vi "Test2_3a_ASIC.vi"(1 "Att. Gain":i32[](array[numeric])=[0, 15], 4 "Voltages comprobation":dbl[](array[numeric])=[0.05, 0.1, 0.2, 0.5, 0.8], 5 "Serial number":string="SN002", 6 "IB_Clip":i32[](array[numeric])=[7, 31, 63], 7 "Save NOW!":bool, 8 "error in":errorcluster, 9 "Cycles Burst":i32=10000, 10 "Channels":i32[](array[numeric])=[0, 1, 2, 3, 4, 5, 6], 11 "Instrument VISA in":T1={"AWG VISA"="generadorpulsos", "Oscilloscope  VISA "="Oscilloscope", "Integration Board IP"="172.16.7.43", "connection ID"=refnum, "report out"=refnum, "report file path"=path "C:/Documents and Settings/CTA_LAB01/Desktop/L0_Asic/L0 Asic Test Data"}) -> (0 "error out":errorcluster={"status"=TRUE, "code"=-1074000000, "source"="Agilent 8000 Series.lvlib:Error Query.vi<ERR>\nInstrument reports:\n-410,\"Query INTERRUPTED\"\r\n0,\"No error\"\r\n\n\n\n<b>Complete call chain:</b>\r\n     Agilent 8000 Series.lvlib:Error Query.vi\r\n     Agilent 8000 Series.lvlib:Close.vi\r\n     Test2_3a_ASIC.vi\r\n     Test_Sum_plus_Maj.vi"}, 3 "Instrument VISA out":T1={"AWG VISA"="generadorpulsos", "Oscilloscope  VISA "="Oscilloscope", "Integration Board IP"="172.16.7.43", "connection ID"=refnum, "report out"=refnum, "report file path"=path "C:/Documents and Settings/CTA_LAB01/Desktop/L0_Asic/L0 Asic Test Data"})   [LabVIEW 2009]
uses:
  <vilib>/Utility/NIReport.llb/NI_report.lvclass
  <vilib>/Utility/NIReport.llb/HTML/NI_HTML.lvclass
  L0_Asic/L0 Asic Test Folder v9/C/Program Files/National Instruments/LabVIEW 2012/instr.lib/Agilent 8000 Series/Public/Configure/Configure Math (Binary Operation).vi
  <instrlib>/Agilent 8000 Series/Public/Data/Read (Multiple Waveforms).vi
  <instrlib>/Agilent 81150/Agilent 81150.lvlib
  L0_Asic/L0 Asic Test Folder v9/C/Program Files/National Instruments/LabVIEW 2012/instr.lib/Agilent 8000 Series/Agilent 8000 Series.lvlib
panel:
  out "dt":dbl
  out "report file path":path=path "C:/Documents and Settings/CTA_LAB01/Desktop/L0_Asic/L0 Asic Test Data"
  in  "Full waveform":bool
  out "Waveform Data":waveform(dbl)[](graph)
  out "time for channel bucle":u32=4294966932
  out "iindex inner bucle":u16=36
  out "time attenuation bucle":u32
  out "points quantity":dbl=10.0
  out "appended array":dbl[](array[numeric])=[9.99999e+37, 9.99999e+37, 2.123674e-09, 7.3101e-11, 0.039346, 0.000993, 2.289694e-09, 1.06004e-10, 1.2407375e-08, 6.2001e-11, 10.0]
  out "read buffer 3":string="V amptd(1),9.99999E+37,9.99999E+37,9.99999E+37,9.99999E+37,9.99999E+37,1.0E+01,+ width(1),2.01719E-09,1.96859E-09,2.19026E-09,2.123674E-09,7.3101E-11,1.0E+01,V amptd(f2),4.065E-02,3.735E-02,4.065E-02,3.9346E-02,9.93E-04,1.0E+01,+ width(f2),2.36565E-09,2.08540E-09,2.47853E-09,2.289694E-09,1.06004E-10,1.0E+01,Time(1-f2),1.236997E-08,1.232364E-08,1.250940E-08,1.2407375E-08,6.2001E-11,1.0E+01\n"
  out "bucle for inner bucle":u32=807
  out "Numeric":i32=185157552
  in  "Clip_sel_b":u32
  in  "Quantity of measurements":u32=100
  in  "End 2":bool
  out "Data output":dbl[][](array[numeric])=[[0.05, 0.0, 0.0, 63.0, 1.0, 9.99999e+37, 9.99999e+37, 2.153239e-09, 8.9127e-11, 0.042394, 0.001347, 2.171806e-09, 1.11555e-10, 1.245617e-08, 7.5484e-11, 10.0, 0.0784, 0.008304761904761905, 0.0], [0.05, 0.0, 0.0, 61.0, 1.0, 9.99999e+37, 9.99999e+37, 2.17591e-09, 7.5138e-11, 0.040364, 0.001353, 2.209888e-09, 7.8523e-11, 1.2524514e-08, 6.7029e-11, 10.0, 0.0784, 0.008304761904761905, 1.0], [0.05, 0.0, 0.0, 59.0, 1.0, 9.99999e+37, 9.99999e+37, 2.193132e-09, 9.3873e-11, 0.04121, 0.001373, 2.164955e-09, 7.7804e-11, 1.2473393e-08, 1.08096e-10, 10.0, 0.0784, 0.008304761904761905, 2.0], [0.05, 0.0, 0.0, 57.0, 1.0, 9.99999e+37, 9.99999e+37, 2.180741e-09, 4.2203e-11, 0.041548, 0.002229, 2.169974e-09, 9.3751e-11, 1.2444116e-08, 5.5272e-11, 11.0, 0.0784, 0.008304761904761905, 3.0], [0.05, 0.0, 0.0, 55.0, 1.0, 9.99999e+37, 9.99999e+37, 2.11229e-09, 3.944e-11, 0.04008, 0.00163, 2.2755e-09, 8.158e-11, 1.245845e-08, 6.277e-11, 9.0, 0.0784, 0.008304761904761905, 4.0], [0.05, 0.0, 0.0, 53.0, 1.0, 9.99999e+37, 9.99999e+37, 2.155237e-09, 6.5891e-11, 0.041291, 0.001559, 2.232596e-09, 7.6359e-11, 1.2466949e-08, 7.7547e-11, 10.0, 0.0784, 0.008304761904761905, 5.0], [0.05, 0.0, 0.0, 7.0, 1.0, 9.99999e+37, 9.99999e+37, 2.12755e-09, 9.1771e-11, 0.03769, 0.001358, 2.349888e-09, 1.38811e-10, 1.2670959e-08, 9.0849e-11, 11.0, 0.0784, 0.008304761904761905, 6.0], [0.05, 0.0, 0.0, 31.0, 1.0, 9.99999e+37, 9.99999e+37, 2.125787e-09, 6.702e-11, 0.039923, 0.00164, 2.260289e-09, 8.9941e-11, 1.2540436e-08, 8.3431e-11, 10.0, 0.0784, 0.008304761904761905, 7.0], [0.05, 0.0, 0.0, 63.0, 1.0, 9.99999e+37, 9.99999e+37, 2.197528e-09, 1.15595e-10, 0.040956, 0.001571, 2.140684e-09, 8.7113e-11, 1.2455007e-08, 4.6485e-11, 10.0, 0.0784, 0.008304761904761905, 8.0], [0.05, 1.0, 0.0, 63.0, 1.0, 9.99999e+37, 9.99999e+37, 2.162133e-09, 7.0698e-11, 0.041207, 0.000752, 2.208266e-09, 1.00999e-10, 1.2372613e-08, 1.00276e-10, 10.0, 0.0784, 0.008304761904761905, 9.0], [0.05, 1.0, 0.0, 61.0, 1.0, 9.99999e+37, 9.99999e+37, 2.13661e-09, 8.2189e-11, 0.039983, 0.00187, 2.265451e-09, 1.14003e-10, 1.2402013e-08, 7.7045e-11, 10.0, 0.0784, 0.008304761904761905, 10.0], [0.05, 1.0, 0.0, 59.0, 1.0, 9.99999e+37, 9.99999e+37, 2.141268e-09, 1.12814e-10, 0.039793, 0.001662, 2.269538e-09, 1.06589e-10, 1.2427868e-08, 8.2834e-11, 10.0, 0.0784, 0.008304761904761905, 11.0], [0.05, 1.0, 0.0, 57.0, 1.0, 9.99999e+37, 9.99999e+37, 2.049403e-09, 8.9792e-11, 0.039527, 0.002147, 2.280746e-09, 1.28958e-10, 1.2384183e-08, 7.0735e-11, 10.0, 0.0784, 0.008304761904761905, 12.0], [0.05, 1.0, 0.0, 55.0, 1.0, 9.99999e+37, 9.99999e+37, 2.164408e-09, 7.8869e-11, 0.041681, 0.001876, 2.182885e-09, 9.6951e-11, 1.2340938e-08, 7.1672e-11, 11.0, 0.0784, 0.008304761904761905, 13.0], [0.05, 1.0, 0.0, 53.0, 1.0, 9.99999e+37, 9.99999e+37, 2.181125e-09, 8.9741e-11, 0.040692, 0.002137, 2.217623e-09, 7.9633e-11, 1.2395418e-08, 1.04033e-10, 10.0, 0.0784, 0.008304761904761905, 14.0], [0.05, 1.0, 0.0, 7.0, 1.0, 9.99999e+37, 9.99999e+37, 2.09233e-09, 6.5939e-11, 0.038027, 0.002128, 2.292623e-09, 1.35118e-10, 1.2538524e-08, 8.874e-11, 10.0, 0.0784, 0.008304761904761905, 15.0], [0.05, 1.0, 0.0, 31.0, 1.0, 9.99999e+37, 9.99999e+37, 2.195349e-09, 8.3233e-11, 0.041018, 0.002034, 2.227655e-09, 8.0651e-11, 1.2425997e-08, 6.1393e-11, 10.0, 0.0784, 0.008304761904761905, 16.0], [0.05, 1.0, 0.0, 63.0, 1.0, 9.99999e+37, 9.99999e+37, 2.150328e-09, 1.0069e-10, 0.040933, 0.00205, 2.19783e-09, 8.0511e-11, 1.2358424e-08, 7.9804e-11, 11.0, 0.0784, 0.008304761904761905, 17.0], [0.05, 2.0, 0.0, 63.0, 1.0, 9.99999e+37, 9.99999e+37, 2.146071e-09, 1.27898e-10, 0.040824, 0.001718, 2.206733e-09, 8.1062e-11, 1.2336427e-08, 5.726e-11, 10.0, 0.0784, 0.008304761904761905, 18.0], [0.05, 2.0, 0.0, 61.0, 1.0, 9.99999e+37, 9.99999e+37, 2.18257e-09, 8.9257e-11, 0.040006, 0.001447, 2.192466e-09, 1.10596e-10, 1.2368096e-08, 6.3926e-11, 10.0, 0.0784, 0.008304761904761905, 19.0], [0.05, 2.0, 0.0, 59.0, 1.0, 9.99999e+37, 9.99999e+37, 2.127276e-09, 7.6459e-11, 0.040334, 0.001234, 2.248995e-09, 1.01211e-10, 1.2365757e-08, 3.5637e-11, 10.0, 0.0784, 0.008304761904761905, 20.0], [0.05, 2.0, 0.0, 57.0, 1.0, 9.99999e+37, 9.99999e+37, 2.126691e-09, 1.01851e-10, 0.041905, 0.001534, 2.214677e-09, 1.14645e-10, 1.2361141e-08, 9.1969e-11, 10.0, 0.0784, 0.008304761904761905, 21.0], [0.05, 2.0, 0.0, 55.0, 1.0, 9.99999e+37, 9.99999e+37, 2.192435e-09, 9.9832e-11, 0.040764, 0.00096, 2.19804e-09, 6.5482e-11, 1.2364743e-08, 9.3874e-11, 10.0, 0.0784, 0.008304761904761905, 22.0], [0.05, 2.0, 0.0, 53.0, 1.0, 9.99999e+37, 9.99999e+37, 2.153844e-09, 6.2552e-11, 0.039026, 0.001388, 2.246022e-09, 9.7907e-11, 1.2344355e-08, 4.8187e-11, 10.0, 0.0784, 0.008304761904761905, 23.0], [0.05, 2.0, 0.0, 7.0, 1.0, 9.99999e+37, 9.99999e+37, 2.218394e-09, 8.2589e-11, 0.037653, 0.001409, 2.315577e-09, 9.9529e-11, 1.2540865e-08, 5.8072e-11, 10.0, 0.0784, 0.008304761904761905, 24.0], [0.05, 2.0, 0.0, 31.0, 1.0, 9.99999e+37, 9.99999e+37, 2.142179e-09, 6.129e-11, 0.040237, 0.001325, 2.255953e-09, 8.6753e-11, 1.2411504e-08, 8.6298e-11, 10.0, 0.0784, 0.008304761904761905, 25.0], [0.05, 2.0, 0.0, 63.0, 1.0, 9.99999e+37, 9.99999e+37, 2.16678e-09, 7.307e-11, 0.03966, 0.00193, 2.25843e-09, 1.2459e-10, 1.238779e-08, 9.08e-11, 9.0, 0.0784, 0.008304761904761905, 26.0], [0.05, 3.0, 0.0, 63.0, 1.0, 9.99999e+37, 9.99999e+37, 2.121706e-09, 9.3892e-11, 0.039916, 0.001529, 2.262652e-09, 7.8947e-11, 1.2388872e-08, 8.2672e-11, 10.0, 0.0784, 0.008304761904761905, 27.0], [0.05, 3.0, 0.0, 61.0, 1.0, 9.99999e+37, 9.99999e+37, 2.182719e-09, 9.6917e-11, 0.038637, 0.001642, 2.243077e-09, 1.01628e-10, 1.2393225e-08, 7.9278e-11, 11.0, 0.0784, 0.008304761904761905, 28.0], [0.05, 3.0, 0.0, 59.0, 1.0, 9.99999e+37, 9.99999e+37, 2.104882e-09, 7.8145e-11, 0.039545, 0.001416, 2.260672e-09, 6.9312e-11, 1.2373319e-08, 5.982e-11, 10.0, 0.0784, 0.008304761904761905, 29.0], [0.05, 3.0, 0.0, 57.0, 1.0, 9.99999e+37, 9.99999e+37, 2.143059e-09, 1.1147e-10, 0.039547, 0.001283, 2.287147e-09, 7.9568e-11, 1.2389127e-08, 5.2602e-11, 11.0, 0.0784, 0.008304761904761905, 30.0], [0.05, 3.0, 0.0, 55.0, 1.0, 9.99999e+37, 9.99999e+37, 2.10482e-09, 6.9561e-11, 0.039043, 0.00127, 2.273205e-09, 8.8457e-11, 1.2378439e-08, 8.4875e-11, 10.0, 0.0784, 0.008304761904761905, 31.0], [0.05, 3.0, 0.0, 53.0, 1.0, 9.99999e+37, 9.99999e+37, 2.166631e-09, 9.2658e-11, 0.039151, 0.000816, 2.302048e-09, 1.32139e-10, 1.2463216e-08, 8.3773e-11, 10.0, 0.0784, 0.008304761904761905, 32.0], [0.05, 3.0, 0.0, 7.0, 1.0, 9.99999e+37, 9.99999e+37, 2.098564e-09, 6.1759e-11, 0.037315, 0.001398, 2.363454e-09, 7.7253e-11, 1.2590485e-08, 6.8209e-11, 10.0, 0.0784, 0.008304761904761905, 33.0], [0.05, 3.0, 0.0, 31.0, 1.0, 9.99999e+37, 9.99999e+37, 2.135125e-09, 7.3789e-11, 0.03888, 0.001329, 2.298536e-09, 5.3729e-11, 1.2501362e-08, 7.0595e-11, 10.0, 0.0784, 0.008304761904761905, 34.0], [0.05, 3.0, 0.0, 63.0, 1.0, 9.99999e+37, 9.99999e+37, 2.123674e-09, 7.3101e-11, 0.039346, 0.000993, 2.289694e-09, 1.06004e-10, 1.2407375e-08, 6.2001e-11, 10.0, 0.0784, 0.008304761904761905, 35.0]]
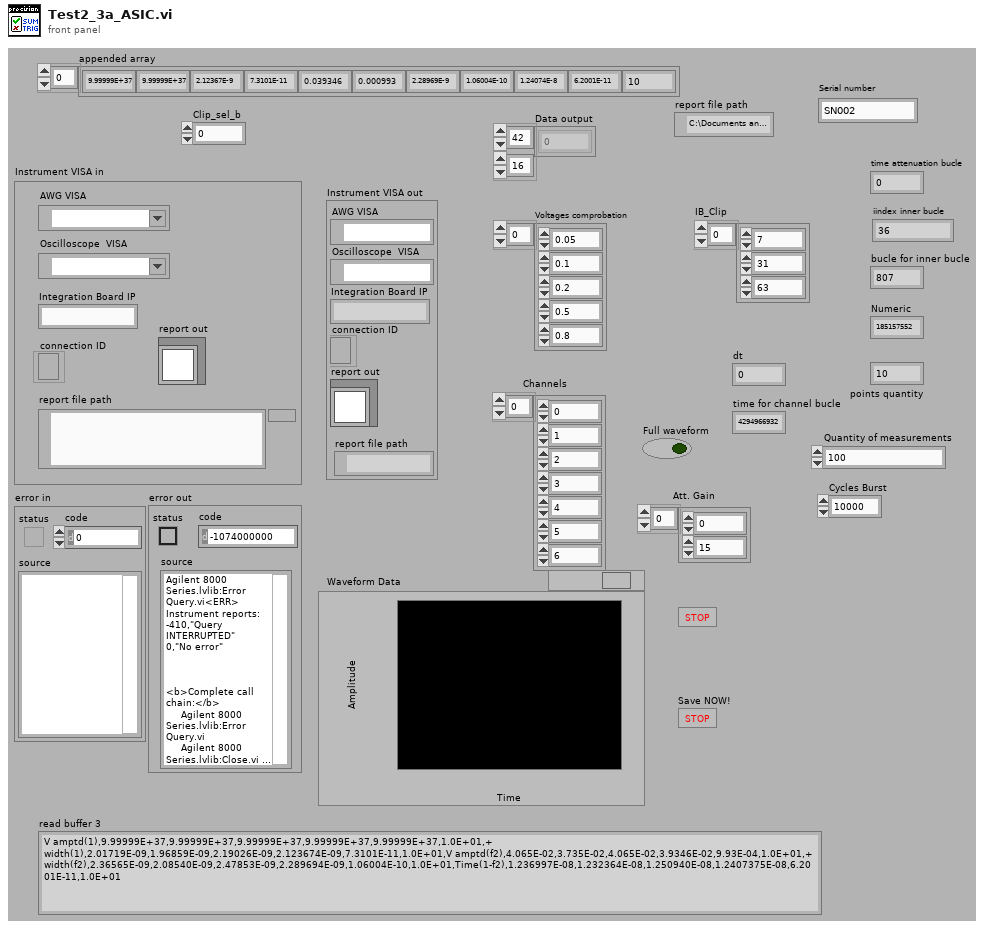
[diagram p1: front panel]
types:
  T1 = cluster{"AWG VISA":refnum<visa-resource-name>, "Oscilloscope  VISA ":refnum<visa-resource-name>, "Integration Board IP":string, "connection ID":refnum<k5>, "report out":refnum<class "NI_report.lvclass">, "report file path":path}
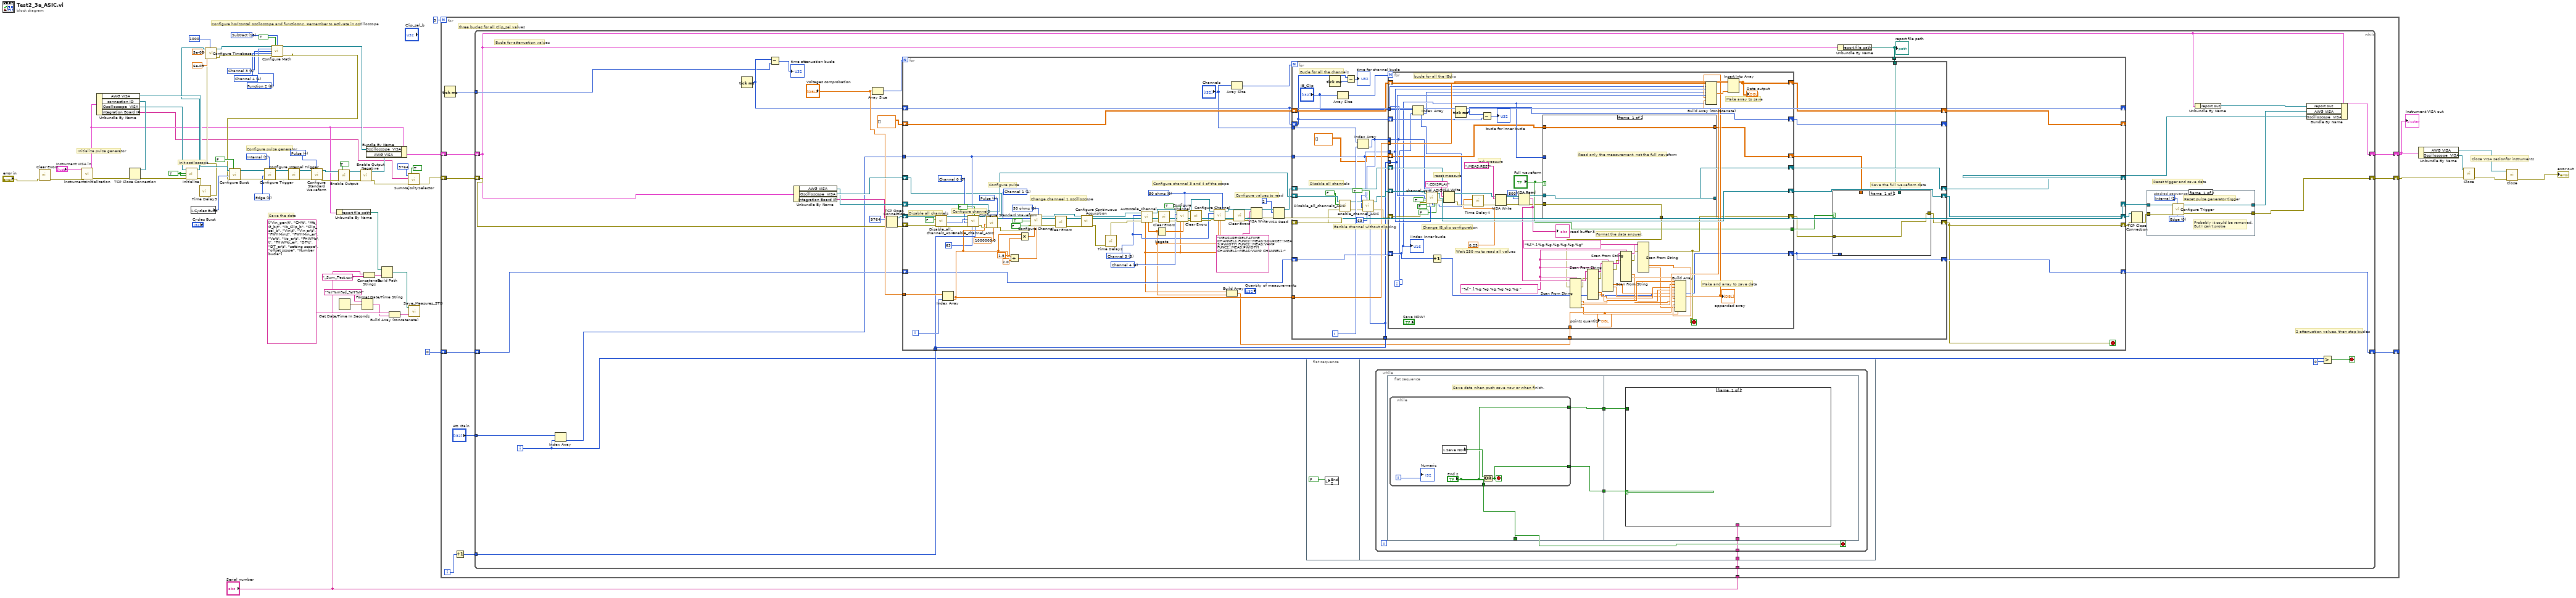
[diagram p0: block diagram]
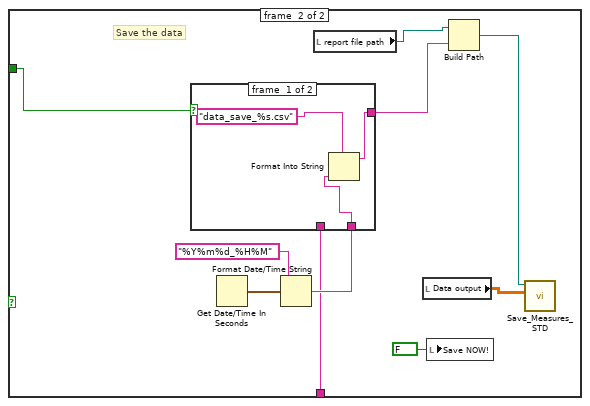
[diagram p2: hidden frame]
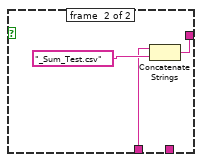
[diagram p3: hidden frame]
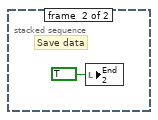
[diagram p4: hidden frame]
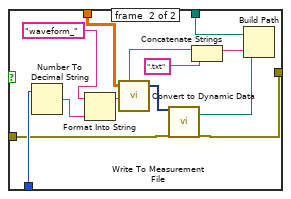
[diagram p5: hidden frame]
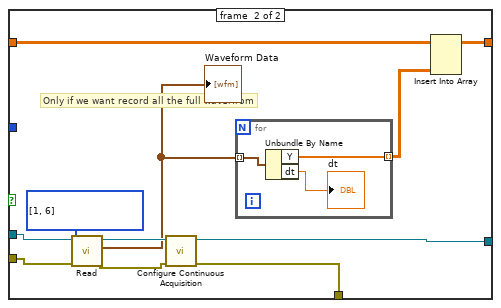
[diagram p6: hidden frame]
diagram:
  w38 = u16 6 items=["Function 1"=5, "Function 2"=6, "Function 3"=7, "Function 4"=8] ("Math Channel (5: Function 1)")
  w42 = u16 15 items=["Add"=12, "Divide"=13, "Multiply"=14, "Subtract"=15, "Common Mode"=16, "Versus"=17] ("Math Operation (12: Add)")
  w37 = 3 items=["Channel 1"=1, "Channel 2"=2, "Channel 3"=3, "Channel 4"=4] ("Channel (1: Channel 1)")
  w36 = 4 items=["Channel 1"=1, "Channel 2"=2, "Channel 3"=3, "Channel 4"=4] ("Channel (1: Channel 1)")
  w57 = u16 1 items=["Immediate", "Internal", "External", "Software Trigger Function"] ("Trigger Source (0: Immediate)")
  w58 = u16 0 items=["Edge", "Level"] ("Trigger Mode (0: Edge)")
  w62 = u16 4 items=["Sine", "Square", "Ramp Up", "Ramp Down", "Pulse", "Noise", "DC"] ("Waveform (0: Sine)")
  w66 = TRUE ("ID Query (True)")
  # "Save the data"
  # "Configure horizontal osciloscope and functio0n2. Remember to activate in oscilloscope"
  # "Close VISA sesionfor instruments"
  # "Configure pulse generator"
  # "Init osciloscope"
  # "Initialize pulse generator"
  n1 = call <vilib>:"Clear Errors.vi"("error in (no error)"="error in") -> ("error out"=w64:errorcluster)  [unwired: 6 in]
  n2 = call "instrumentsInitialization.vi"("error in"=w64, "Instrument VISA in"="Instrument VISA in") -> ("error out"=w51:errorcluster, "Instrument VISA out"=w10:T1)  [unwired: 8 in]
  n3 = Unbundle By Name(w10) -> ("AWG VISA"=w47:refnum<visa-resource-name>, "connection ID"=w52:refnum<k5>, "Oscilloscope  VISA"=w48:refnum<visa-resource-name>, "Integration Board IP"=w1:string)
  n4 = TCP Close Connection(connection ID=w52, error in (no error)=w51) -> (error out=w7:errorcluster)  [unwired: 1 in, 1 out]
  n5 = call <instrlib>:"Initialize.vi"("error in (no error)"=w7, "Reset (True)"=w66, "ID Query (True)"=w66, "VISA resource name"=w48) -> ("error out"=w65:errorcluster, "VISA resource name out"=w35:refnum<visa-resource-name>)  [unwired: 6 in]
  n6 = local read "Cycles Burst"() -> (w61:i32)
  n7 = call "Time Delay3"("error in (no error)"=w65) -> ("error out"=w34:errorcluster)  [unwired: 10 in]
  n8 = call <instrlib>:"Configure Timebase.vi"("Record Length (1000)"=1000, "error in (no error)"=w34, "Position (0.0 s)"=6e-09, "Timebase (0.005 s)"=5e-08, "VISA resource name"=w35) -> ("error out"=w39:errorcluster, "VISA resource name out"=w40:refnum<visa-resource-name>)  [unwired: 5 in]
  n9 = call-poly "Configure Math.vi"("VISA resource name"=w40, "Enable Math Channel (T:Enable)"=TRUE, "Math Operation (12: Add)"=w42, "Math Channel (5: Function 1)"=w38, "Math Operand (1: Channel 1)"=w37, "Math Operand (2: Channel 2)"=w36, "error in (no error)"=w39) -> ("VISA resource name out"=w23:refnum<visa-resource-name>, "error out"=w24:errorcluster)  [unwired: 7 in]
  n10 = call <instrlib>:"Configure Burst.vi"("Enable Burst (F: Disable)"=FALSE, "error in (no error)"=w24, "Burst Count (2)"=w61, "VISA resource name"=w47) -> ("error out"=w60:errorcluster, "VISA resource name out"=w59:refnum<visa-resource-name>)  [unwired: 6 in]
  n11 = call <instrlib>:"Configure Trigger.vi"("Trigger Source (0: Immediate)"=w57, "error in (no error)"=w60, "Trigger Mode (0: Edge)"=w58, "VISA resource name"=w59) -> ("error out"=w56:errorcluster, "VISA resource name out"=w55:refnum<visa-resource-name>)  [unwired: 6 in]
  n12 = call <instrlib>:"Configure Internal Trigger.vi"("error in (no error)"=w56, "VISA resource name"=w55) -> ("error out"=w53:errorcluster, "VISA resource name out"=w54:refnum<visa-resource-name>)  [unwired: 8 in]
  n13 = call <instrlib>:"Configure Standard Waveform.vi"("Waveform (0: Sine)"=w62, "error in (no error)"=w53, "VISA resource name"=w54) -> ("error out"=w46:errorcluster, "VISA resource name out"=w45:refnum<visa-resource-name>)  [unwired: 7 in]
  n14 = Unbundle By Name(w10) -> ("report file path"=w9:path)
  n15 = call <instrlib>:"Enable Output.vi"("Enable Output (T: Enable)"=TRUE, "error in (no error)"=w46, "VISA resource name"=w45) -> ("error out"=w21:errorcluster, "VISA resource name out"=w20:refnum<visa-resource-name>)  [unwired: 7 in]
  n16 = Get Date/Time In Seconds() -> (seconds since 1Jan1904=w15:timestamp)
  n17 = call <instrlib>:"Enable Output Negative.vi"("error in (no error)"=w21, "VISA resource name"=w20) -> ("error out"=w4:errorcluster, "VISA resource name out"=w19:refnum<visa-resource-name>)  [unwired: 8 in]
  n18 = Format Date/Time String(time format string (%c)="%Y%m%d_%H%M", seconds (now)=w15) -> (date/time string=w13:string)  [unwired: 1 in]
  n19 = Concatenate Strings("Serial number", "_Sum_Test.csv" ("format string")) -> (w11:string)
  n20 = Bundle By Name(cluster=w10, "Oscilloscope  VISA"=w23, "AWG VISA"=w19) -> (w26:T1)
  n21 = Build Path(base path=w9, name or relative path=w11) -> (appended path=w18:path)
  n22 = Build Array (concatenate)(string[] ["Vin_gen\t", "CH\t", "Att_G_b\t", "Ib_Clip_b", "Clip_sel_b", "Vin\t", "Vin er\t", "FWHMin\t", "FWHMin_er", "Vo\t", "Vo_er\t", "FHWMo\t", "FHWMo_er", "DT\t", "DT_er\t", "setting scope", "offset scope", "Number bucle"] ("appended array"), w13) -> (w16:string[])
  n23 = call "SumMajoritySelector.vi"("On Sum\nOff Majority"=TRUE, "error in (no error)"=w4, "address"=w1, "remote port or service name"=u16 9764) -> ("error out"=w3:errorcluster)  [unwired: 7 in]
  n24 = call "Save_Measures_STD.vi"("appended array"=w16, "file path (dialog if empty)"=w18) -> ()  [unwired: 10 in]
  n25 = for {
    N: 3 -> [_]
    shift-right: [w77] -> w29
    shift-left: w3 -> [w73]
    shift-right: [w76] -> w27
    shift-left: w26 -> [w72]
    shift-right: [w69] -> _
    shift-left: u16 0 ("remote port or service name") -> [w70]
    tunnel: "Serial number" -> [w68]
    i -> [w74]
    # "three bucles for all Clip_sel values"
    n26 = Tick Count (ms)() -> (millisecond timer value=w71:u32)
    n27 = Increment(x=w74) -> (x+1=w75:i32)
    n28 = while {
      shift-right: [w83] -> w77
      shift-left: w73 -> [w99]
      shift-right: [w106] -> w76
      shift-left: w72 -> [w86]
      tunnel: w75 -> [w81]
      tunnel: w71 -> [w91]
      shift-right: [w89] -> w69
      shift-left: w70 -> [w90]
      tunnel: w68 -> [w82]
      tunnel: "Att. Gain" -> [w80]
      i -> [w79]
      stop <- w108 stop-if-true
      # "2 attenuation values, then stop bucles"
      # "Reset trigger and save data"
      # "Bucle for attenuation values"
      n29 = Index Array(array=w80, index=w79) -> (element=w78:i32)
      n30 = Tick Count (ms)() -> (millisecond timer value=w92:u32)
      n31 = Subtract(x=w92, y=w91) -> (x-y=→"time attenuation bucle":u32)
      n32 = Unbundle By Name(w86) -> ("AWG VISA"=w103:refnum<visa-resource-name>, "Oscilloscope  VISA"=w104:refnum<visa-resource-name>, "Integration Board IP"=w100:string)
      n33 = Array Size(array="Voltages comprobation") -> (size(s)=w109:i32)
      n34 = TCP Open Connection(address=w100, remote port or service name=u16 9764, error in (no error)=w99) -> (connection ID=w94:refnum<k5>, error out=w98:errorcluster)  [unwired: 2 in]
      n35 = flat-sequence {
        tunnel: w82 -> [w112]
        frame #0 {
          n36 = local write "End 2"(FALSE ("End")) -> ()
        }
        frame #1 {
          n37 = while {
            tunnel: w112 -> [w113]
            stop <- w114 stop-if-true
            n38 = flat-sequence {
              tunnel: [w119] -> w116
              tunnel: [w118] -> w115
              tunnel: [w117] -> w114
              tunnel: w116 -> [w126]
              tunnel: w115 -> [w125]
              tunnel: w113 -> [w124]
              frame #0 {
                # "Save data when push save now or when finish."
                n39 = while {
                  tunnel: [w122] -> w119
                  tunnel: ["End 2"] -> w118
                  tunnel: ["End 2"] -> w117
                  i -> [w121]
                  stop <- w122 stop-if-true
                  n40 = local read "Save NOW!"() -> (w123:bool)
                  n41 = Or(x=w123, y="End 2") -> (x .or. y?=w122:bool)
                  "Numeric" <- w121
                }
              }
              frame #1 {
                n42 = case shown="True" w126 {
                  tunnel: w125 -> [_ w133]
                  tunnel: w124 -> [_ w127]
                  frame #0 {
                  }
                  frame #1 {
                    # "Save the data"
                    n43 = Get Date/Time In Seconds() -> (seconds since 1Jan1904=w131:timestamp)
                    n44 = Format Date/Time String(time format string (%c)="%Y%m%d_%H%M", seconds (now)=w131) -> (date/time string=w129:string)  [unwired: 1 in]
                    n45 = case shown="True" w133 {
                      tunnel: [w138 w141] -> w132
                      tunnel: w129 -> [w137 _]
                      tunnel: w127 -> [_ w140]
                      frame #0 {
                        n46 = Format Into String(format string="data_save_%s.csv", w137) -> (resulting string=w138:string)  [unwired: 2 in, 1 out]
                      }
                      frame #1 {
                        n47 = Concatenate Strings(w140, "_Sum_Test.csv" ("format string")) -> (w141:string)
                      }
                    }
                    n48 = local read "report file path"() -> (w128:path)
                    n49 = local read "Data output"() -> (w135:dbl[][])
                    n50 = local write "Save NOW!"(FALSE ("Save NOW!")) -> ()
                    n51 = Build Path(base path=w128, name or relative path=w132) -> (appended path=w136:path)
                    n52 = call "Save_Measures_STD.vi"("Data in"=w135, "file path (dialog if empty)"=w136) -> ()  [unwired: 10 in]
                  }
                }
              }
            }
          }
        }
      }
      n53 = Unbundle By Name(w86) -> ("report file path"=w85:path)
      "report file path" <- w85
      n54 = for {
        N: w109 -> [_]
        shift-right: [w150] -> w96
        shift-left: w98 -> [w182]
        shift-right: [w210] -> _
        shift-left: dbl[][] [] -> [w211]
        tunnel: "Voltages comprobation" -> [w209]
        shift-right: [w170] -> w105
        shift-left: w103 -> [w217]
        shift-right: [w203] -> w87
        shift-left: w104 -> [w187]
        tunnel: w78 -> [w198]
        tunnel: w81 -> [w195]
        shift-right: [w181] -> w95
        shift-left: w94 -> [w180]
        shift-right: [w153] -> _
        shift-left: w92 -> [w153]
        shift-right: [w152] -> w89
        shift-left: w90 -> [w166]
        tunnel: w85 -> [w151]
        i -> [w216]
        stop <- w150 stop-if-true
        w159 = 3 items=["Channel 1"=1, "Channel 2"=2, "Channel 3"=3, "Channel 4"=4] ("Channel (1: Channel 1)")
        w183 = 4 items=["Channel 1"=1, "Channel 2"=2, "Channel 3"=3, "Channel 4"=4] ("Channel (1: Channel 1)")
        w160 = u32 0 items=["50 ohms", "1 Mohms"] ("Input Impedance (1: 1 Mohms)")
        w194 = u16 0 items=["Channel 0", "Channel 1", "Channel 2", "Channel 3", "Channel 4", "Channel 5", "Channel 6"] ("Channel")
        w213 = u32 0 items=["50 ohms", "1 Mohms"] ("Input Impedance (1: 1 Mohms)")
        w215 = 1 items=["Channel 1"=1, "Channel 2"=2, "Channel 3"=3, "Channel 4"=4] ("Channel (1: Channel 1)")
        w218 = u16 4 items=["Sine", "Square", "Ramp Up", "Ramp Down", "Pulse", "Noise", "DC"] ("Waveform (0: Sine)")
        # "Configure values to read"
        # "Configure channel 3 and 4 of the scope"
        # "Change channeel 1 oscilloscope"
        # "Configure pulse"
        # "Configure channel0"
        # "Disable all channels"
        n55 = call "Disable_all_channels_ASIC.vi"("error in"=w182, "Clip_en_b"=FALSE, "connection ID"=w180) -> ("error out"=w201:errorcluster, "id_out"=w199:i32, "connection ID out"=w200:refnum<k5>)  [unwired: 6 in]
        n56 = Index Array(array=w209, index=w216) -> (element=w193:dbl)
        n57 = call "enable_channel_ASIC.vi"("Clip_sel_b"=w195, "maj/sum"=TRUE, "Ib_clipVb"=u32 63, "Att gain"=w198, "error in"=w201, "Channel"=w194, "id_in"=w199, "connection ID"=w200) -> ("error out"=w202:errorcluster, "connection ID out"=w172:refnum<k5>)  [unwired: 1 in, 1 out]
        n58 = call <instrlib>:"Configure Standard Waveform.vi"("Frequency (1000.0 Hz)"=1000000.0, "Waveform (0: Sine)"=w218, "error in (no error)"=w202, "Amplitude (1.0 Vpp)"=w193, "VISA resource name"=w217) -> ("error out"=w188:errorcluster, "VISA resource name out"=w170:refnum<visa-resource-name>)  [unwired: 5 in]
        n59 = Divide(x=w193, y=2.0) -> (x/y=w197:dbl)
        n60 = Multiply(x=w193, y=1.5) -> (x*y=w191:dbl)
        n61 = call "Configure Channel.vi"("VISA resource name"=w187, "Enable Channel (Enable)"=TRUE, "BW Limit 20MHz (Disable)"=FALSE, "Input Impedance (1: 1 Mohms)"=w213, "Channel (1: Channel 1)"=w215, "error in (no error)"=w188, "Vertical Range (2.0 V)"=w191, "Vertical Offset (0.0 V)"=w197) -> ("VISA resource name out"=w186:refnum<visa-resource-name>, "error out"=w185:errorcluster)  [unwired: 6 in]
        n62 = call <vilib>:"Clear Errors.vi"("error in (no error)"=w185) -> ("error out"=w184:errorcluster)  [unwired: 6 in]
        n63 = call "Configure Continuous Acquisition.vi"("error in (no error)"=w184, "VISA resource name"=w186) -> ("error out"=w196:errorcluster, "VISA resource name out"=w178:refnum<visa-resource-name>)  [unwired: 8 in]
        n64 = call "Time Delay2"("error in (no error)"=w196) -> ("error out"=w179:errorcluster)  [unwired: 10 in]
        n65 = call "Autoscale_Channel.vi"("error in"=w179, "Channel"=w159, "VISA resource name"=w178) -> ("error out"=w204:errorcluster, "VISA resource name out"=w207:refnum<visa-resource-name>, "Offset"=w158:dbl, "VerticalRange"=w157:dbl)  [unwired: 5 in]
        n66 = Negate(x=w158) -> (-x=w189:dbl)
        n67 = call <vilib>:"Clear Errors.vi"("error in (no error)"=w204) -> ("error out"=w205:errorcluster)  [unwired: 6 in]
        n68 = call "Configure Channel.vi"("VISA resource name"=w207, "Enable Channel (Enable)"=TRUE, "Input Impedance (1: 1 Mohms)"=w160, "Channel (1: Channel 1)"=w183, "error in (no error)"=w205, "Vertical Range (2.0 V)"=w157, "Vertical Offset (0.0 V)"=w189) -> ("VISA resource name out"=w162:refnum<visa-resource-name>, "error out"=w206:errorcluster)  [unwired: 7 in]
        n69 = call <vilib>:"Clear Errors.vi"("error in (no error)"=w206) -> ("error out"=w164:errorcluster)  [unwired: 6 in]
        n70 = call "Configure Channel.vi"("VISA resource name"=w162, "Input Impedance (1: 1 Mohms)"=w160, "Channel (1: Channel 1)"=w159, "error in (no error)"=w164, "Vertical Range (2.0 V)"=w157, "Vertical Offset (0.0 V)"=w158) -> ("VISA resource name out"=w161:refnum<visa-resource-name>, "error out"=w165:errorcluster)  [unwired: 8 in]
        n71 = Build Array(w157, w158) -> (w190:dbl[])
        n72 = Array Size(array="Channels") -> (size(s)=w171:i32)
        n73 = call <vilib>:"Clear Errors.vi"("error in (no error)"=w165) -> ("error out"=w163:errorcluster)  [unwired: 6 in]
        n74 = VISA Write(VISA resource name=w161, write buffer="MEASURE:DELTATIME CHANNEL1,FUNC2;:MEAS:SOURCE?;:MEAS:PWIDTH FUNC2;:MEAS:VAMP FUNC2;:MEAS:PWIDTH CHANNEL1;:MEAS:VAMP CHANNEL1;", error in (no error)=w163) -> (VISA resource name out=w177:refnum<visa-resource-name>, error out=w176:errorcluster)  [unwired: 1 out]
        n75 = VISA Read(VISA resource name=w177, byte count=u32 2, error in (no error)=w176) -> (VISA resource name out=w173:refnum<visa-resource-name>, error out=w174:errorcluster)  [unwired: 2 out]
        n76 = for {
          N: w171 -> [_]
          tunnel: w198 -> [w228]
          tunnel: w195 -> [w235]
          tunnel: w193 -> [w251]
          tunnel: w190 -> [w250]
          shift-right: [w253] -> w210
          shift-left: w211 -> [w254]
          shift-right: [w252] -> w203
          shift-left: w173 -> [w248]
          shift-right: [w249] -> w181
          shift-left: w172 -> [w241]
          shift-right: [w226] -> w150
          shift-left: w174 -> [w243]
          tunnel: "Channels" -> [w247]
          shift-right: [w222] -> w152
          shift-left: w166 -> [w245]
          shift-right: [w229] -> _
          shift-left: w153 -> [w230]
          tunnel: w151 -> [w224]
          i -> [w246]
          # "Eanble channel without clipping"
          # "Disable all channels"
          # "Save the full wavefrom data"
          # "Bucle for all the channels"
          n77 = Tick Count (ms)() -> (millisecond timer value=w231:u32)
          n78 = Array Size(array="IB_Clip") -> (size(s)=w233:i32)
          n79 = call "Disable_all_channels_ASIC.vi"("error in"=w243, "Clip_en_b"=FALSE, "connection ID"=w241) -> ("error out"=w244:errorcluster, "connection ID out"=w239:refnum<k5>)  [unwired: 6 in, 1 out]
          n80 = Subtract(x=w230, y=w231) -> (x-y=→"time for channel bucle":u32)
          n81 = Index Array(array=w247, index=w246) -> (element=w236:i32)
          n82 = call "enable_channel_ASIC.vi"("Clip_sel_b"=w235, "maj/sum"=TRUE, "Ib_clipVb"=u32 63, "Att gain"=w228, "error in"=w244, "Channel"=w236, "connection ID"=w239) -> ("error out"=w242:errorcluster, "connection ID out"=w240:refnum<k5>)  [unwired: 2 in, 1 out]
          n83 = for {
            N: w233 -> [_]
            shift-right: [w274] -> w225
            shift-left: w242 -> [w299]
            tunnel: w251 -> [w331]
            shift-right: [w312] -> w253
            shift-left: w254 -> [w329]
            tunnel: w228 -> [w326]
            shift-right: [w277] -> w252
            shift-left: w248 -> [w301]
            tunnel: w235 -> [w325]
            shift-right: [w327] -> w249
            shift-left: w240 -> [w328]
            tunnel: w250 -> [w323]
            shift-right: [w321] -> w229
            shift-left: w230 -> [w322]
            tunnel: w236 -> [w282]
            shift-right: [w281] -> w222
            shift-left: w245 -> [w275]
            tunnel: "IB_Clip" -> [w280]
            shift-right: [w272] -> w223
            shift-left: dbl[][] [] ("Y") -> [w273]
            tunnel: ["Full waveform"] -> w227
            i -> [w269]
            stop <- w274 stop-if-true
            w294 = "%[^,],%g,%g,%g,%g,%g,%g," ("format string")
            # "Make and array to save data"
            # "Wait 250 ms to read all values"
            # "Change IB_clip configuration"
            # "Make array to save"
            # "Format the data answer."
            # "ask measure"
            # "reset measure"
            # "bucle for all the IBclip"
            n84 = Index Array(array=w280, index=w269) -> (element=w268:i32)
            n85 = call "channel_conf_ASIC.vi"("connection ID"=w328, "Ring"=w282, "Clip_sel_b"=w325, "CompBuf_en_b"=TRUE, "error out"=w299, "Att gain"=w326, "Ib_ClipVb"=w268, "Clip_en_b"=FALSE, "Att_en_b"=FALSE) -> ("connection ID out"=w327:refnum<k5>, "error out 2"=w297:errorcluster)  [unwired: 2 in, 3 out]
            n86 = Increment(x=w275) -> (x+1=w281:u16)
            n87 = VISA Write(VISA resource name=w301, write buffer=":CDISPLAY", error in (no error)=w297) -> (VISA resource name out=w303:refnum<visa-resource-name>, error out=w296:errorcluster)  [unwired: 1 out]
            n88 = Tick Count (ms)() -> (millisecond timer value=w321:u32)
            n89 = call "Time Delay4"("error in (no error)"=w296, "Delay Time (s)"=0.25 ("x*y")) -> ("error out"=w314:errorcluster)  [unwired: 9 in]
            n90 = Subtract(x=w321, y=w322) -> (x-y=→"bucle for inner bucle":u32)
            n91 = VISA Write(VISA resource name=w303, write buffer=":MEAS:RES?", error in (no error)=w314) -> (VISA resource name out=w319:refnum<visa-resource-name>, error out=w318:errorcluster)  [unwired: 1 out]
            n92 = VISA Read(VISA resource name=w319, byte count=u32 800, error in (no error)=w318) -> (VISA resource name out=w278:refnum<visa-resource-name>, read buffer=w315:string, error out=w279:errorcluster)  [unwired: 1 out]
            "read buffer 3" <- w315
            n93 = case shown="False" "Full waveform" {
              tunnel: w279 -> [w334 w343]
              tunnel: w278 -> [w333 w345]
              tunnel: [w333 w341] -> w277
              tunnel: [w334 w335] -> w276
              tunnel: w275 -> [_ _]
              tunnel: w273 -> [w332 w338]
              tunnel: [w332 w337] -> w272
              frame #0 {
                # "Read only the measurement, not the full waveform"
              }
              frame #1 {
                w344 = i32[] [1, 6] items=["Channel 1"=1, "Channel 2"=2, "Channel 3"=3, "Channel 4"=4, "Function 1"=5, "Function 2"=6, "Function 3"=7, "Function 4"=8, "Memory 1"=9, "Memory 2"=10, "Memory 3"=11, "Memory 4"=12] ("Channels")
                # "Only if we want record all the full waverfrom"
                n94 = call-poly "Read.vi"("error in (no error)"=w343, "Channels"=w344, "VISA resource name"=w345) -> ("error out"=w340:errorcluster, "Waveform Data"=w339:waveform(dbl)[], "VISA resource name out"=w342:refnum<visa-resource-name>)  [unwired: 6 in]
                "Waveform Data" <- w339
                n95 = call "Configure Continuous Acquisition.vi"("error in (no error)"=w340, "VISA resource name"=w342) -> ("error out"=w335:errorcluster, "VISA resource name out"=w341:refnum<visa-resource-name>)  [unwired: 8 in]
                n96 = for {
                  tunnel: w339 -> [w348] mode=indexing
                  tunnel: [w347] -> w336 mode=indexing
                  n97 = Unbundle By Name(w348) -> ("Y"=w347:dbl[], "dt"=→"dt":dbl)
                }
                n98 = Insert Into Array(array=w338, new element=w336) -> (w337:dbl[][])  [unwired: 2 in]
              }
            }
            n99 = Scan From String(format string=w294, input string=w315, error in=w276) -> (remaining string=w311:string, error out=w304:errorcluster, output 5=w293:dbl, output 6=w291:dbl, output 7=w292:dbl)  [unwired: 12 in, 1 out]
            "points quantity" <- w292
            n100 = Scan From String(format string=w294, input string=w311, error in=w304) -> (remaining string=w308:string, error out=w305:errorcluster, output 5=w290:dbl, output 6=w289:dbl)  [unwired: 13 in, 1 out]
            n101 = Scan From String(format string=w294, input string=w308, error in=w305) -> (remaining string=w309:string, error out=w306:errorcluster, output 5=w288:dbl, output 6=w287:dbl)  [unwired: 13 in, 1 out]
            n102 = Scan From String(format string=w294, input string=w309, error in=w306) -> (remaining string=w310:string, error out=w307:errorcluster, output 5=w286:dbl, output 6=w285:dbl)  [unwired: 13 in, 1 out]
            n103 = Scan From String(format string="%[^,],%g,%g,%g,%g,%g,%g", input string=w310, error in=w307) -> (error out=w274:errorcluster, output 5=w284:dbl, output 6=w283:dbl)  [unwired: 13 in, 2 out]
            n104 = Build Array(w293, w291, w290, w289, w288, w287, w286, w285, w284, w283, w292) -> (w313:dbl[])
            "appended array" <- w313
            n105 = Build Array (concatenate)(w331, w282, w326, w268, w325, w313, w323, w275) -> (w330:dbl[])
            n106 = Insert Into Array(array=w329, new element=w330) -> (w312:dbl[][])  [unwired: 2 in]
            "Data output" <- w312
            "iindex inner bucle" <- w275
          }
          n107 = case shown="True" w227 {
            tunnel: w223 -> [_ w267]
            tunnel: w225 -> [w255 w257]
            tunnel: [w255 w265] -> w226
            tunnel: w224 -> [_ w259]
            tunnel: w222 -> [_ w258]
            frame #0 {
            }
            frame #1 {
              n108 = Number To Decimal String(number=w258) -> (decimal integer string=w264:string)  [unwired: 1 in]
              n109 = Format Into String(initial string="waveform_", w264) -> (resulting string=w262:string)  [unwired: 2 in, 1 out]
              n110 = call "Convert to Dynamic Data"("2D Array"=w267) -> ("Dynamic Data Type"=w266:dynamicdata)  [unwired: 3 in]
              n111 = Concatenate Strings(w262, ".txt" ("string")) -> (w256:string)
              n112 = Build Path(base path=w259, name or relative path=w256) -> (appended path=w260:path)
              n113 = call "Write To Measurement File"("Signals"=w266, "error in (no error)"=w257, "Filename"=w260) -> ("error out"=w265:errorcluster)  [unwired: 14 in, 2 out]
            }
          }
        }
      }
      n114 = TCP Close Connection(connection ID=w95, error in (no error)=w96) -> (error out=w97:errorcluster)  [unwired: 1 in, 1 out]
      n115 = stacked-sequence {
        tunnel: w97 -> [w146 _]
        tunnel: [w145 _] -> w83
        tunnel: w105 -> [w144 _]
        tunnel: [w143 _] -> w88
        frame #0 {
          w147 = u16 1 items=["Immediate", "Internal", "External", "Software Trigger Function"] ("Trigger Source (0: Immediate)")
          w148 = u16 0 items=["Edge", "Level"] ("Trigger Mode (0: Edge)")
          # "Probably it could be removed. \nBut I can't probe"
          # "Reset pulse generator tirgger"
          n116 = call <instrlib>:"Configure Trigger.vi"("Trigger Source (0: Immediate)"=w147, "error in (no error)"=w146, "Trigger Mode (0: Edge)"=w148, "VISA resource name"=w144) -> ("error out"=w145:errorcluster, "VISA resource name out"=w143:refnum<visa-resource-name>)  [unwired: 6 in]
        }
        frame #1 {
          # "Save data"
          n117 = local write "End 2"(TRUE ("End 2")) -> ()
        }
      }
      n118 = Unbundle By Name(w86) -> ("report out"=w84:refnum<class "NI_report.lvclass">)
      n119 = Bundle By Name(cluster=w86, "report out"=w84, "AWG VISA"=w88, "Oscilloscope  VISA"=w87) -> (w106:T1)
      n120 = Greater?(x=w79, y=0) -> (0:w108:bool)
    }
  }
  "Instrument VISA out" <- w27
  n121 = Unbundle By Name(w27) -> ("AWG VISA"=w30:refnum<visa-resource-name>, "Oscilloscope  VISA"=w31:refnum<visa-resource-name>)
  n122 = call <instrlib>:"Close.vi"("error in (no error)"=w29, "VISA resource name"=w31) -> ("error out"=w32:errorcluster)  [unwired: 9 in]
  n123 = call <instrlib>:"Close.vi"("error in (no error)"=w32, "VISA resource name"=w30) -> ("error out"=→"error out":errorcluster)  [unwired: 9 in]
